vi "DataTreeCtrl moveData.vi"(8 "error in (no error)":errorcluster, 10 "moveParam":T1, 11 "DataTreeCtrl in":refnum<class "DataTreeCtrl.lvclass">) -> (0 "error out":errorcluster, 2 "accepted":bool, 3 "DataTreeCtrl out":refnum<class "DataTreeCtrl.lvclass">)   [LabVIEW 2018, in "DataTreeCtrl.lvclass"]
uses:
  DataTreeCtrl.lvclass
  ctl/FMstateMachineEnum.ctl
  DataTreeCtrl.lvclass/DataTreeCtrl.ctl
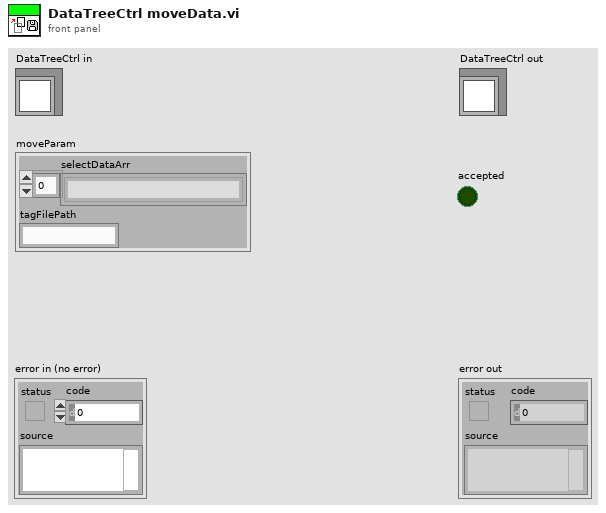
[diagram p1: front panel]
types:
  T1 = cluster{"selectDataArr":string[], "tagFilePath":string}
  T2 = typedef "FMstateMachineEnum.ctl" = enum16{"none", "init", "openTDMS", "closeTDMS", "getDataList", "getDataInfo", "getTimeStamp", "getCurrPath", "getRemark", "overwriteRemark", "readData", "deleteData", "moveData"}
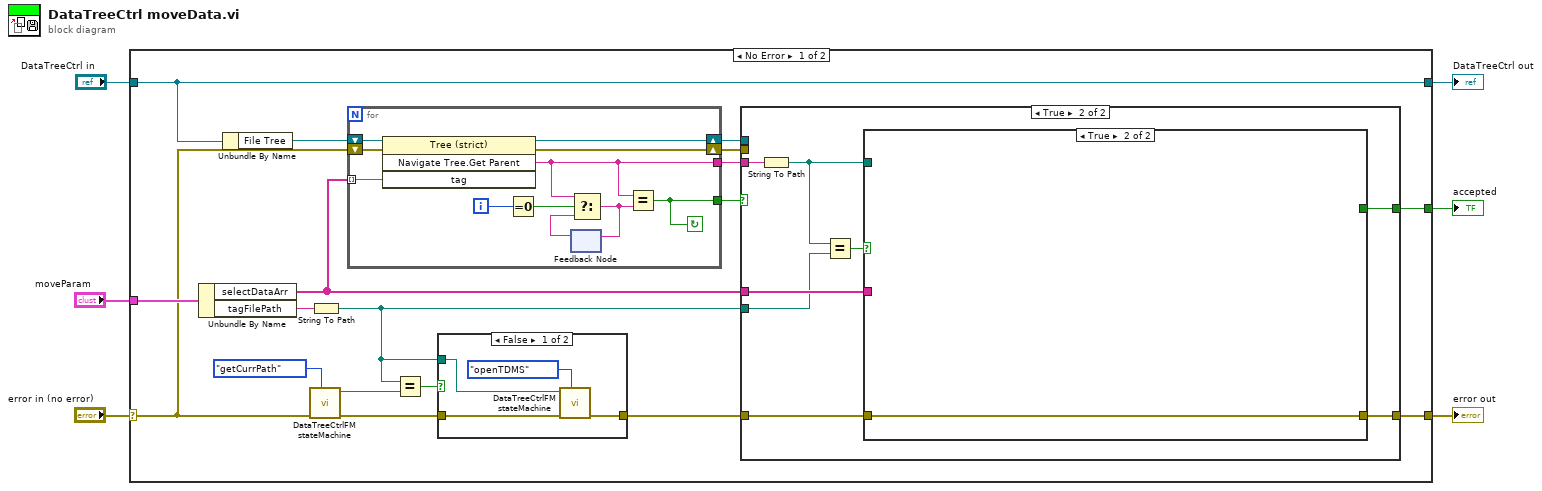
[diagram p0: block diagram]
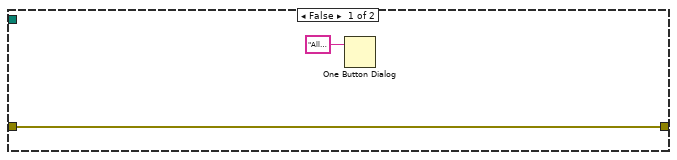
[diagram p3: hidden frame]
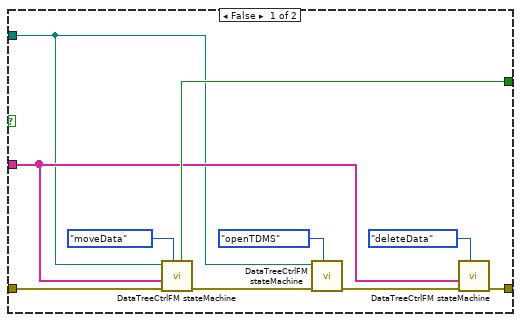
[diagram p4: hidden frame]
diagram:
  n1 = case shown="No Error" "error in (no error)" {
    selector: "error in (no error)" -> [w8 w63]
    tunnel: [w9 w63] -> w5
    tunnel: [w23 w62] -> w3
    tunnel: "DataTreeCtrl in" -> [w23 w62]
    tunnel: "moveParam" -> [w24 _]
    tunnel: [w10 _] -> w1
    frame No Error {
      n2 = Unbundle By Name(w24) -> ("selectDataArr"=w18:string[], "tagFilePath"=w15:string)
      n3 = Unbundle By Name(w23) -> ("File Tree"=w22:refnum<vi>)
      n4 = call "DataTreeCtrlFM stateMachine.vi"("Func"=FMstateMachineEnum."getCurrPath", "error in (no error)"=w8) -> ("error out"=w12:errorcluster, "tdmsFilePath out"=w14:path)  [unwired: 4 in, 4 out]
      n5 = String To Path(string=w15) -> (path=w7:path)
      n6 = for {
        tunnel: w18 -> [w61] mode=indexing
        tunnel: [w56] -> w21
        shift-right: [w54] -> w20
        shift-left: w22 -> [w55]
        shift-right: [w53] -> w19
        shift-left: w8 -> [w52]
        tunnel: [w51] -> w17
        i -> [w60]
        stop <- w56 continue-if-true
        n7 = invoke class="Tree (strict)" method="Navigate Tree.Get Parent"(reference=w55, error in=w52, "tag"=w61) -> (reference out=w54:refnum<vi>, error out=w53:errorcluster, "Navigate Tree:Get Parent"=w51:string)  [unwired: 1 in, 1 out]
        n8 = Equal To 0?(x=w60) -> (x = 0?=w59:bool)
        n9 = feedback #1() -> (w58:string)  [unwired: 1 in]
        n10 = Select(t=w51, s=w59, f=w58) -> (s? t:f=w57:string)
        n11 = feedback-in #1(w57) -> ()
        n12 = Equal?(x=w51, y=w57) -> (x = y?=w56:bool)
      }
      n13 = Equal?(x=w7, y=w14) -> (x = y?=w13:bool)
      n14 = case shown="False" w13 {
        tunnel: w12 -> [w27 w29]
        tunnel: [w26 w29] -> w11
        tunnel: w7 -> [w25 _]
        frame False {
          n15 = call "DataTreeCtrlFM stateMachine.vi"("Func"=FMstateMachineEnum."openTDMS", "error in (no error)"=w27, "tdmsFilePath in"=w25) -> ("error out"=w26:errorcluster)  [unwired: 3 in, 5 out]
        }
        frame True {
        }
      }
      n16 = case shown="True" w21 {
        tunnel: w20 -> [_ _]
        tunnel: w19 -> [_ _]
        tunnel: w18 -> [_ w36]
        tunnel: w17 -> [_ w37]
        tunnel: w11 -> [w30 w38]
        tunnel: [_ w39] -> w10
        tunnel: [w30 w35] -> w9
        tunnel: w7 -> [_ w33]
        frame False {
          n17 = One Button Dialog(message="Allow only single file to single file.") -> ()  [unwired: 1 in, 1 out]
        }
        frame True {
          n18 = String To Path(string=w37) -> (path=w34:path)
          n19 = Equal?(x=w34, y=w33) -> (x = y?=w32:bool)
          n20 = case shown="True" w32 {
            tunnel: [w48 _] -> w39
            tunnel: w38 -> [w47 w50]
            tunnel: w36 -> [w42 _]
            tunnel: [w41 w50] -> w35
            tunnel: w34 -> [w40 _]
            frame False {
              n21 = call "DataTreeCtrlFM stateMachine.vi"("Func"=FMstateMachineEnum."moveData", "error in (no error)"=w47, "multiDatasName"=w42, "tdmsFilePath in"=w40) -> ("error out"=w45:errorcluster, "valid"=w48:bool)  [unwired: 2 in, 4 out]
              n22 = call "DataTreeCtrlFM stateMachine.vi"("Func"=FMstateMachineEnum."openTDMS", "error in (no error)"=w45, "tdmsFilePath in"=w40) -> ("error out"=w43:errorcluster)  [unwired: 3 in, 5 out]
              n23 = call "DataTreeCtrlFM stateMachine.vi"("Func"=FMstateMachineEnum."deleteData", "error in (no error)"=w43, "multiDatasName"=w42) -> ("error out"=w41:errorcluster)  [unwired: 3 in, 5 out]
            }
            frame True {
            }
          }
        }
      }
    }
    frame Error {
    }
  }
  "error out" <- w5
  "DataTreeCtrl out" <- w3
  "accepted" <- w1
